vi "AUTON_Init.vi"(11 "Default File":i32) -> (0 "Auton Array":dbl[][](array[numeric]) format="%0.3f", 1 "Current File":string, 2 "Auton Files":string[](array[string]), 3 "Number of Auton Files":i64)   [LabVIEW 2011]
uses:
  <vilib>/Rock Robotics/WPI/DriverStation/DriverStationLCD/WPI_DriverStationLCDLCDLine.ctl
  <vilib>/Utility/file.llb/Read From Spreadsheet File (DBL).vi
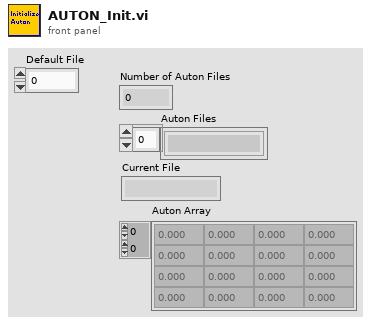
[diagram p1: front panel]
types:
  T1 = typedef "WPI_DriverStationLCDLCDLine.ctl" = enum16{"Main - Line 1", "User - Line 2", "User - Line 3", "User - Line 4", "User - Line 5", "User - Line 6"}
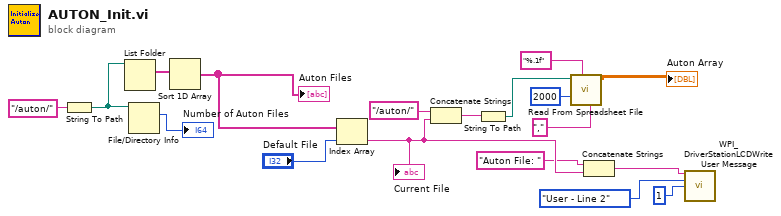
[diagram p0: block diagram]
diagram:
  n1 = String To Path(string="/auton/") -> (path=w4:path)
  n2 = List Folder(path=w4) -> (filenames=w5:string[])  [unwired: 1 in, 5 out]
  n3 = File/Directory Info(path=w4) -> (size=→"Number of Auton Files":i64)  [unwired: 1 in, 6 out]
  n4 = Sort 1D Array(array=w5) -> (sorted array=w7:string[])
  "Auton Files" <- w7
  n5 = Index Array(array=w7, index="Default File") -> (element=w18:string)
  "Current File" <- w18
  n6 = Concatenate Strings("/auton/" ("string"), w18) -> (w14:string)
  n7 = String To Path(string=w14) -> (path=w13:path)
  n8 = call-poly <vilib>:"Read From Spreadsheet File.vi"("delimiter (\\t)"="," ("delimiter (\\t)"), "format (%.3f)"="%.1f", "number of rows (all:-1)"=2000, "file path (dialog if empty)"=w13) -> ("all rows"=→"Auton Array":dbl[][])  [unwired: 1 in, 6 out]
  n9 = Concatenate Strings("Auton File: ", w18) -> (w11:string)
  n10 = call <vilib>:"WPI_DriverStationLCDWrite User Message.vi"("line text"=w11, "line"=WPI_DriverStationLCDLCDLine."User - Line 2", "starting column"=i8 1) -> ()  [unwired: 2 in, 11 out]
